vi "Get File Type.vi"(11 "App Data In":T1) -> (2 "FileType":T2, 3 "App Data Out":T1)   [LabVIEW 2019]
uses:
  TypeDef/File Type.ctl
  TypeDef/App Data.ctl
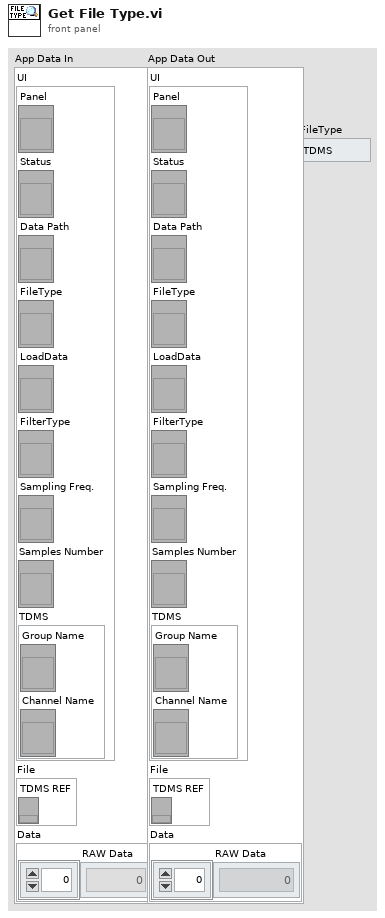
[diagram p1: front panel]
types:
  T1 = typedef "App Data.ctl" = cluster{"UI":cluster{"Panel":refnum<vi>, "Status":refnum<vi>, "Data Path":refnum<vi>, "FileType":refnum<vi>, "LoadData":refnum<vi>, "FilterType":refnum<vi>, "Sampling Freq.":refnum<vi>, "Samples Number":refnum<vi>, "TDMS":cluster{"Group Name":refnum<vi>, "Channel Name":refnum<vi>}}, "File":cluster{"TDMS REF":refnum<k34>}, "Data":cluster{"RAW Data":dbl[]}}
  T2 = typedef "File Type.ctl" = enum32{"TDMS", "CSV"}
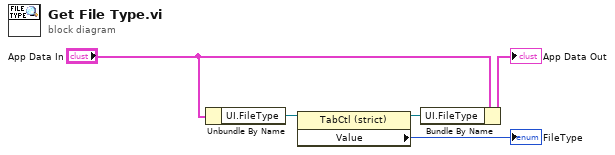
[diagram p0: block diagram]
diagram:
  n1 = Unbundle By Name("App Data In") -> ("UI.FileType"=w4:refnum<vi>)
  n2 = property class="TabCtl (strict)"(reference=w4) -> (reference out=w5:refnum<vi>, "Value"=→"FileType":enum32{"TDMS", "CSV"})  [unwired: 1 in, 1 out]
  n3 = Bundle By Name(cluster="App Data In", "UI.FileType"=w5) -> (→"App Data Out":T1)
